vi "Ensure Default CellStyleFormat.vi"(8 "error in":errorcluster, 11 "SpreadsheetDoc in":refnum<k24>) -> (0 "error out":errorcluster, 3 "SpreadsheetDoc out":refnum<k24>)   [LabVIEW 2019, in "Open Xml.lvlib"]
uses:
  Open Xml.lvlib
  D:/git/Open-Xml-LabVIEW/Source/DocumentFormat.OpenXml.dll
  DocumentFormat.OpenXml.dll
  D:/git/Open-Xml-LabVIEW/Source/DocumentFormat.OpenXml.Framework.dll
  DocumentFormat.OpenXml.Framework.dll
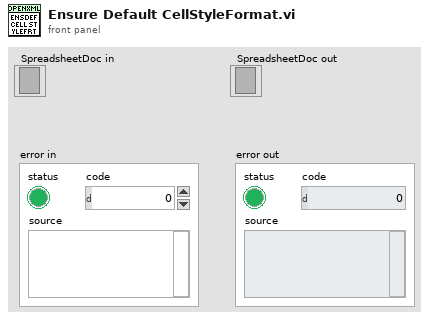
[diagram p1: front panel]
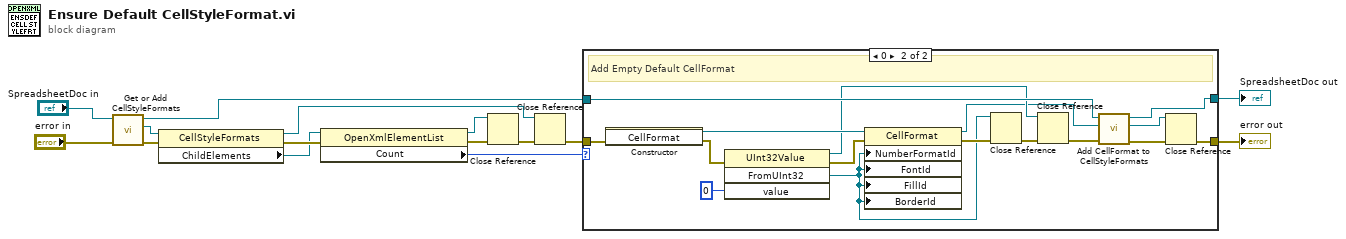
[diagram p0: block diagram]
diagram:
  n1 = call "Get or Add CellStyleFormats.vi"("error in"="error in", "SpreadsheetDoc in"="SpreadsheetDoc in") -> ("error out"=w11:errorcluster, "CellStyleFormats"=w10:refnum<k24>, "SpreadsheetDoc out"=w7:refnum<k24>)  [unwired: 7 in]
  n2 = property class="CellStyleFormats"(reference=w10, error in=w11) -> (reference out=w2:refnum<k24>, error out=w9:errorcluster, "ChildElements"=w4:refnum<k24>)
  n3 = property class="OpenXmlElementList"(reference=w4, error in=w9) -> (reference out=w1:refnum<k24>, error out=w6:errorcluster, "Count"=w8:i32)
  n4 = Close Reference(reference=w1, error in (no error)=w6) -> (error out=w5:errorcluster)
  n5 = Close Reference(reference=w2, error in (no error)=w5) -> (error out=w3:errorcluster)
  n6 = case shown="0" w8 {
    tunnel: w7 -> [w16 w33]
    tunnel: w3 -> [w17 w32]
    tunnel: [w17 w29] -> w14
    tunnel: [w16 w31] -> w15
    frame Default {
      # "Default"
    }
    frame 0 {
      # "Add Empty Default CellFormat"
      n7 = constructor class="CellFormat"(error in=w32) -> (reference out=w26:refnum<k24>, error out=w22:errorcluster)  [unwired: 2 in, 1 out]
      n8 = invoke class="UInt32Value" method="FromUInt32"(error in=w22, "value"=u32 0) -> (reference out=w24:refnum<k24>, error out=w21:errorcluster, "FromUInt32"=w18:refnum<k24>)  [unwired: 2 in, 1 out]
      n9 = property class="CellFormat"(reference=w26, error in=w21, "NumberFormatId"=w18, "FontId"=w18, "FillId"=w18, "BorderId"=w18) -> (reference out=w20:refnum<k24>, error out=w27:errorcluster)
      n10 = Close Reference(reference=w18, error in (no error)=w27) -> (error out=w19:errorcluster)
      n11 = Close Reference(reference=w24, error in (no error)=w19) -> (error out=w25:errorcluster)
      n12 = call "Add CellFormat to CellStyleFormats.vi"("error in"=w25, "CellFormat in"=w20, "SpreadsheetDoc in"=w33) -> ("error out"=w30:errorcluster, "CellFormat out"=w28:refnum<k24>, "SpreadsheetDoc out"=w31:refnum<k24>)  [unwired: 5 in, 1 out]
      n13 = Close Reference(reference=w28, error in (no error)=w30) -> (error out=w29:errorcluster)
    }
  }
  "SpreadsheetDoc out" <- w15
  "error out" <- w14
